vi "HRTF-Register Device Dialog Events.vi"(7 "Refs":refnum<vi>[](array[refnum]), 11 "error in (no error)":errorcluster) -> (8 "Event Registration Refnum":refnum<event-registration>, 15 "error out":errorcluster)   [LabVIEW 2020]
uses:
  Utility VIs/Controls/KTable/KTable.xctl
  Utility VIs/Controls/KTable/Events.ctl
  Utility VIs/Controls/KTable/Event Data.ctl
  Utility VIs/Controls/KTable/Event Type.ctl
panel:
  in  "temp":cluster{"OutputTable":T1, "InputTable":T1}
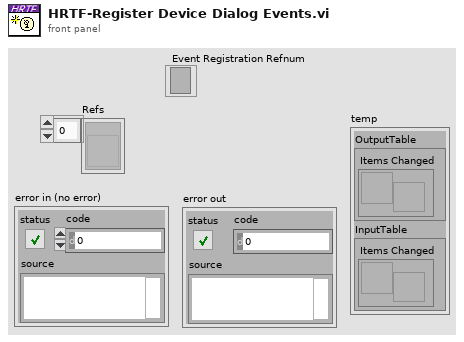
[diagram p1: front panel]
types:
  T1 = typedef "KTable.xctl/Events.ctl" = cluster{"Items Changed":refnum<user-event>}
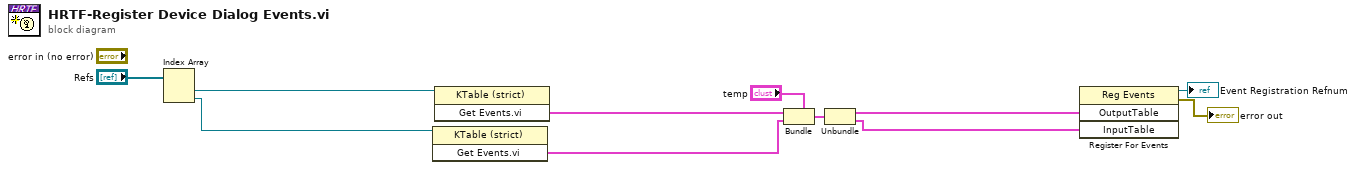
[diagram p0: block diagram]
diagram:
  n1 = Index Array(array="Refs") -> (element #1=w8:refnum<vi>, element #2=w6:refnum<vi>)  [unwired: 2 in]
  n2 = invoke on="Invoke Node" class="KTable (strict)" method="Get Events.vi"(reference=w6) -> ("Get Events.vi"=w5:T1)  [unwired: 2 in, 2 out]
  n3 = invoke on="Invoke Node" class="KTable (strict)" method="Get Events.vi"(reference=w8) -> ("Get Events.vi"=w7:T1)  [unwired: 2 in, 2 out]
  n4 = Bundle(cluster="temp", "OutputTable"=w7, "InputTable"=w5) -> (w11:cluster{"OutputTable":T1, "InputTable":T1})
  n5 = Unbundle(w11) -> ("OutputTable"=w4:T1, "InputTable"=w3:T1)
  n6 = register-events(w4, w3) -> (reference out=→"Event Registration Refnum":refnum<event-registration>, error out=→"error out":errorcluster)  [unwired: 2 in]
